vi "mqttTCPIPbrokerConnect.vi"(0 "mqtt in":refnum<class "mqtt.lvclass">, 11 "error in (no error)":errorcluster) -> (4 "mqtt out":refnum<class "mqtt.lvclass">, 15 "error out":errorcluster)   [LabVIEW 2021, in "mqtt.lvclass"]
uses:
  mqtt.lvclass
  mqtt.lvclass/mqtt.ctl
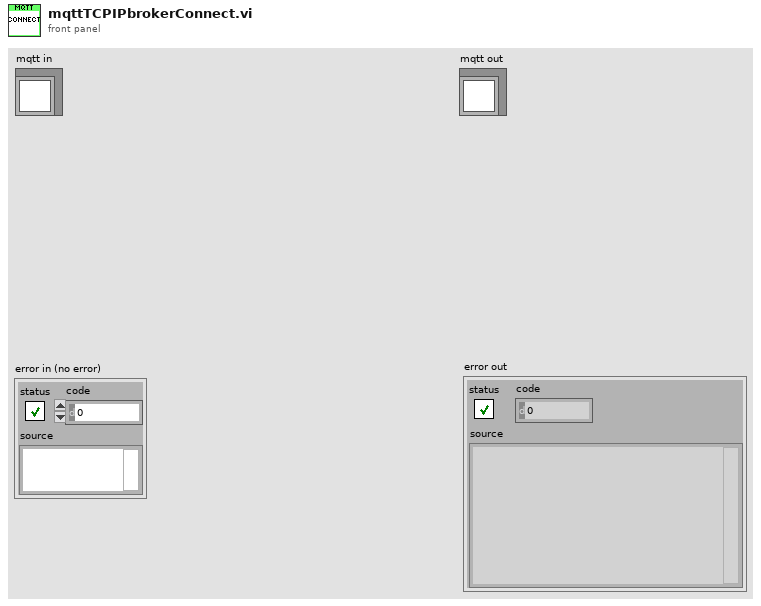
[diagram p1: front panel]
types:
  T1 = typedef "mqttBroker.ctl" = cluster{"IP or  URL of the broker":string, "connTimeout":i32, "writeTimeout":i32, "readTimeout":i32, "subTimeout":i32, "Port":u16}
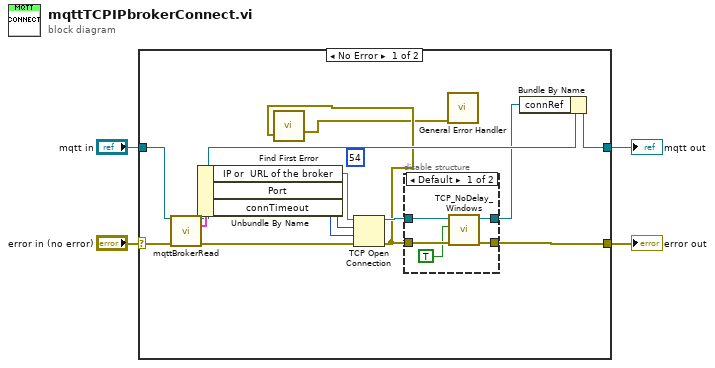
[diagram p0: block diagram]
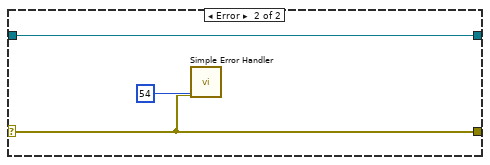
[diagram p3: hidden frame]
diagram:
  n1 = case shown="No Error" "error in (no error)" {
    selector: "error in (no error)" -> [w16 w26]
    tunnel: [w17 w26] -> w1
    tunnel: [w7 w28] -> w2
    tunnel: "mqtt in" -> [w11 w28]
    frame No Error {
      (unwired) 54 ("error code (no error:0)")
      n2 = call "mqttBrokerRead.vi"("mqtt in"=w11, "error in (no error)"=w16) -> ("mqtt out"=w9:refnum<class "mqtt.lvclass">, "broker"=w14:T1, "error out"=w15:errorcluster)  [unwired: 11 in]
      n3 = Unbundle By Name(w14) -> ("IP or  URL of the broker"=w13:string, "Port"=w12:u16, "connTimeout"=w10:i32)
      n4 = TCP Open Connection(address=w13, remote port or service name=w12, timeout ms (60000)=w10, error in (no error)=w15) -> (connection ID=w18:refnum<k5>, error out=w6:errorcluster)  [unwired: 1 in]
      n5 = call <vilib>:"Find First Error.vi"("error in (no error)"=w6) -> ("error out"=w5:errorcluster)  [unwired: 3 in, 1 out]
      n6 = disable-structure shown="Default" {
        disable-tunnel: w18 -> [w23 w25]
        disable-tunnel: w6 -> [w22 w24]
        disable-tunnel: [w21 w24] -> w17
        disable-tunnel: [w19 w25] -> w8
        frame condition #0 (active) {
          n7 = call "TCP_NoDelay_Windows.vi"("error in (no error)"=w22, "TCP_NODELAY (true)"=TRUE, "connID"=w23) -> ("error out"=w21:errorcluster, "connID 2"=w19:refnum<k5>)  [unwired: 3 in]
        }
        frame condition #1 {
        }
      }
      n8 = call <vilib>:"General Error Handler.vi"("error in (no error)"=w5) -> ()  [unwired: 10 in, 5 out]
      n9 = Bundle By Name(cluster=w9, "connRef"=w8) -> (w7:refnum<class "mqtt.lvclass">)
    }
    frame Error {
      n10 = call <vilib>:"Simple Error Handler.vi"("error code (no error:0)"=54, "error in (no error)"=w26) -> ()  [unwired: 3 in, 5 out]
    }
  }
  "error out" <- w1
  "mqtt out" <- w2
